vi "Error 8001 incomplete data.vi"() -> (3 "error out":errorcluster)   [LabVIEW 2018, in "Frame Analizer.lvclass"]
uses:
  Frame Analizer.lvclass
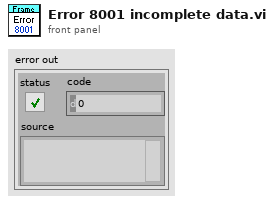
[diagram p1: front panel]
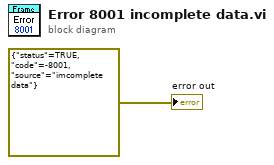
[diagram p0: block diagram]
diagram:
  "error out" <- errorcluster {"status"=TRUE, "code"=-8001, "source"="imcomplete data"} ("error out")
